vi "aceleracion.vi"(11 "a0":dbl) -> (3 "Real Matrix":T1)   [LabVIEW 2018]
uses:
  <vilib>/Analysis/Matrix/Datatypes/RealMatrix.ctl
  <vilib>/Analysis/Matrix/NI_Matrix.lvlib
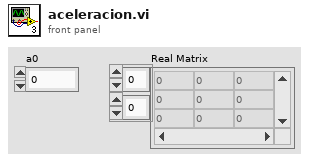
[diagram p1: front panel]
types:
  T1 = typedef "NI_Matrix.lvlib/RealMatrix.ctl" = dbl[][]
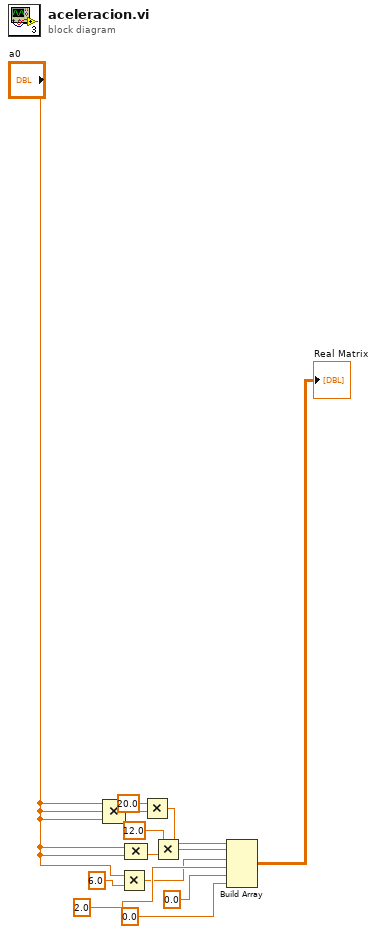
[diagram p0: block diagram]
diagram:
  n1 = Compound Arithmetic op=MULTIPLY("a0", "a0", "a0") -> (w2:dbl)
  n2 = Multiply(x="a0", y=6.0 ("x")) -> (x*y=w9:dbl)
  n3 = Compound Arithmetic op=MULTIPLY("a0", "a0") -> (w5:dbl)
  n4 = Multiply(x=20.0, y=w2) -> (x*y=w3:dbl)
  n5 = Multiply(x=12.0, y=w5) -> (x*y=w7:dbl)
  n6 = Build Array(w3, w7, w9, 2.0 ("y"), 0.0, 0.0) -> (→"Real Matrix":T1)
